vi "1 - Offline client lifecycle.vi"() -> ()   [LabVIEW 2020]
uses:
  client/client.lvlib
panel:
  out "function return 2":i32
  out "function return":i32
  out "buf out":string
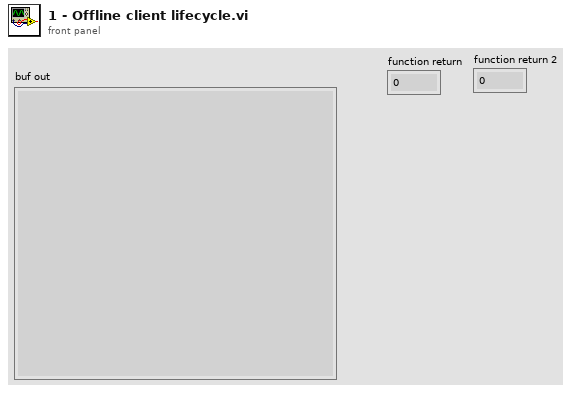
[diagram p1: front panel]
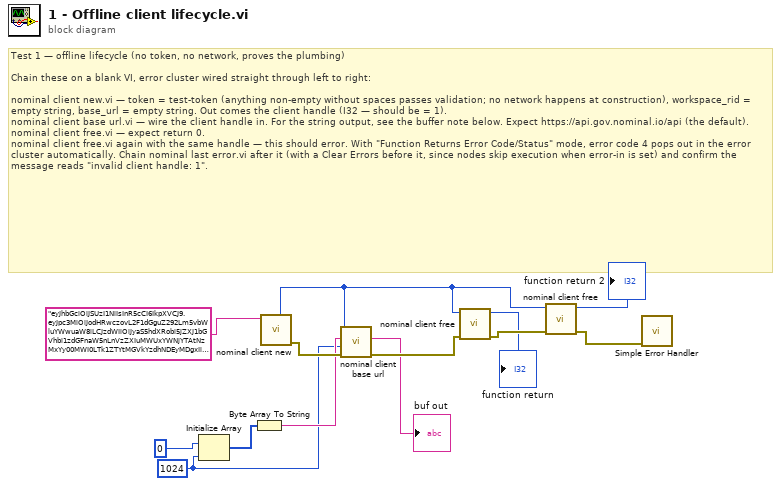
[diagram p0: block diagram]
diagram:
  w2 = 1024
  # "Test 1 — offline lifecycle (no token, no network, proves the plumbing)\n\nChain these on a blank VI, error cluster wired straight through left to right:\n\nnominal client new.vi — token = test-token (anything non-empty without spaces passes validation; no network happens at construction), workspace_rid = empty string, base_url = empty string. Out comes the client handle (I32 — should be = 1).\nnominal client base url.vi — wire the client handle in. For the string output, see the buffer note below. Expect https://api.gov.nominal.io/api (the default).\nnominal client free.vi — expect return 0.\nnominal client free.vi again with the same handle — this should error. With \"Function Returns Error Code/Status\" mode, error code 4 pops out in the error cluster automatically. Chain nominal last error.vi after it (with a Clear Errors before it, since nodes skip execution when error-in is set) and confirm the message reads \"invalid client handle: 1\"."
  n1 = Initialize Array(u8 0, w2) -> (w1:u8[])
  n2 = Byte Array To String(unsigned byte array=w1) -> (string=w4:string)
  n3 = call "nominal client new.vi"("token"="eyJhbGciOiJSUzI1NiIsInR5cCI6IkpXVCJ9.eyJpc3MiOiJodHRwczovL2F1dGguZ292Lm5vbWluYWwuaW8iLCJzdWIiOiJyaS5hdXRobi5jZXJ1bGVhbi1zdGFnaW5nLnVzZXIuMWUxYWNjYTAtNzMxYy00MWI0LTk1ZTYtMGVkYzdhNDEyMDgxIiwibm9taW5hbCI6eyJ1c2VyX3V1aWQiOiIxZTFhY2NhMC03MzFjLTQxYjQtOTVlNi0wZWRjN2E0MTIwODEiLCJvcmdhbml6YXRpb25fdXVpZCI6IjdkODAyZDRlLTdmMWMtNDViOS1iYTA1LWY3ZjYzMjM1MDRkNiIsInNjb3BlIjpbIlRydWVTY29wZSIsIklOU1RBTkNFIl19LCJleHAiOjE3ODYyMTg5MzEsImF1ZCI6Imh0dHBzOi8vYXBpLmdvdi5ub21pbmFsLmlvIn0.b1R-OTsEoXRBlxRscJn3Ag9EOYiyqHQjGKv9pTBUhInJclWOAX28gvJz6cmUxBR8ljVp-rSapiHV0CRGFIIfuFzaXlOXcd2GntvPqV_t5DapkDu1kJ_iQYTfrrD3NJUE9koxTrQHBzkmhIsGH21lGLaq9QIc0FltD4EptmGRrGEB99Q3zXbogZFfbscLU9-j1OiblutRKnsmUv2SOjkWYxjMdhkNGo9NB-b5njzqYCn1Mr8s0p7PsnblL-QoPUUUEMQgUzGOgtDotBPYajRze-E-Tir02zbfpKdple5wSNXtveaNR1N9fXXWzJleehOcnRYrykIDFXTw7A8GnLvJvQ") -> ("error out"=w12:errorcluster, "out_client out"=w13:i32)  [unwired: 8 in, 1 out]
  n4 = call "nominal client base url.vi"("error in (no error)"=w12, "cap"=w2, "buf"=w4, "client"=w13) -> ("error out"=w11:errorcluster, "buf out"=→"buf out":string)  [unwired: 4 in, 2 out]
  n5 = call "nominal client free.vi"("error in (no error)"=w11, "client"=w13) -> ("error out"=w10:errorcluster, "function return"=→"function return":i32)  [unwired: 8 in]
  n6 = call "nominal client free.vi"("error in (no error)"=w10, "client"=w13) -> ("error out"=w7:errorcluster, "function return"=→"function return 2":i32)  [unwired: 8 in]
  n7 = call <vilib>:"Simple Error Handler.vi"("error in (no error)"=w7) -> ()  [unwired: 4 in, 5 out]
